vi "Read Visa.vi"(8 "error in (no error)":errorcluster, 10 "Read":bool, 11 "UI Actor in":refnum<class "UI Actor.lvclass">) -> (0 "error out":errorcluster, 3 "UI Actor out":refnum<class "UI Actor.lvclass">)   [LabVIEW 2020, in "UI Actor.lvlib" / "UI Actor.lvclass"]
uses:
  UI Actor.lvclass
  UI Actor.lvclass/UI Actor.ctl
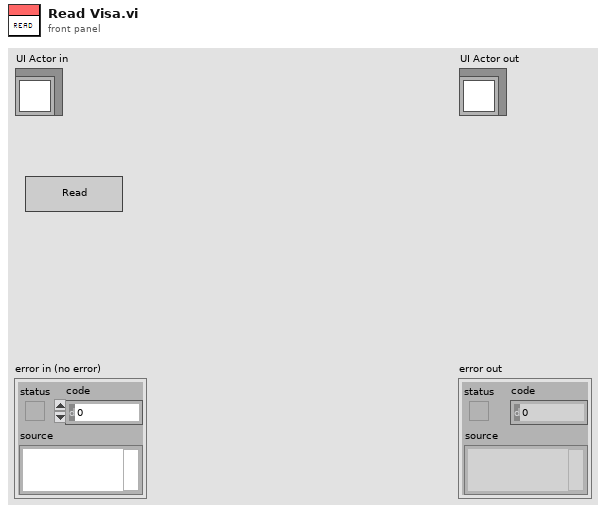
[diagram p1: front panel]
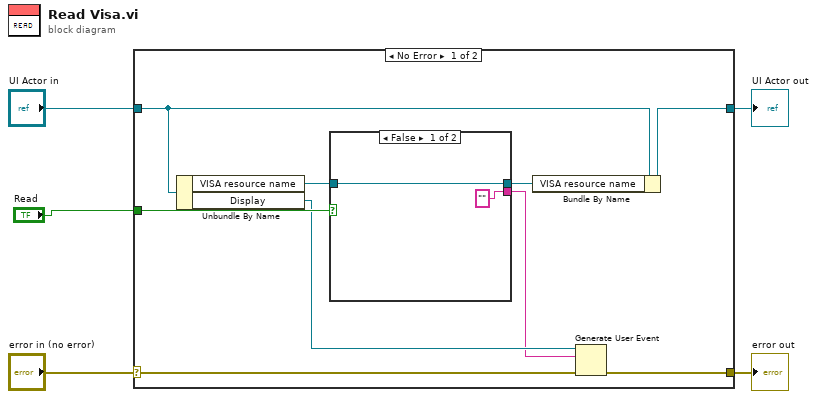
[diagram p0: block diagram]
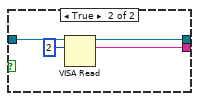
[diagram p2: hidden frame]
diagram:
  n1 = case shown="No Error" "error in (no error)" {
    selector: "error in (no error)" -> [w14 w22]
    tunnel: [w8 w22] -> w4
    tunnel: [w10 w21] -> w2
    tunnel: "UI Actor in" -> [w12 w21]
    tunnel: "Read" -> [w13 _]
    frame No Error {
      n2 = Unbundle By Name(w12) -> ("VISA resource name"=w11:refnum<visa-resource-name>, "Display"=w7:refnum<user-event>)
      n3 = case shown="False" w13 {
        tunnel: w11 -> [w15 w20]
        tunnel: [w15 w18] -> w9
        tunnel: ["" ("read buffer") w17] -> w6
        frame False {
        }
        frame True {
          n4 = VISA Read(VISA resource name=w20, byte count=u32 2) -> (VISA resource name out=w18:refnum<visa-resource-name>, read buffer=w17:string)  [unwired: 1 in, 2 out]
        }
      }
      n5 = Bundle By Name(cluster=w12, "VISA resource name"=w9) -> (w10:refnum<class "UI Actor.lvclass">)
      n6 = Generate User Event(user event=w7, event data cluster=w6, error in=w14) -> (error out=w8:errorcluster)  [unwired: 1 in, 1 out]
    }
    frame Error {
    }
  }
  "error out" <- w4
  "UI Actor out" <- w2
